vi "Generate Simulated DI Data.vi"(8 "error in":errorcluster, 11 "IONames[]":string[](array[string])) -> (0 "error out":errorcluster, 1 "timestamp":dbl, 2 "data":bool[](array[boolean]))   [LabVIEW 2017, in "DAQ.lvclass"]
doc: "Developed by Kevin Thompson\nkevin@thompsonengineering.net\n\nCopyright 2018-2020\nThompson Engineering, LLC"
uses:
  DAQ.lvclass
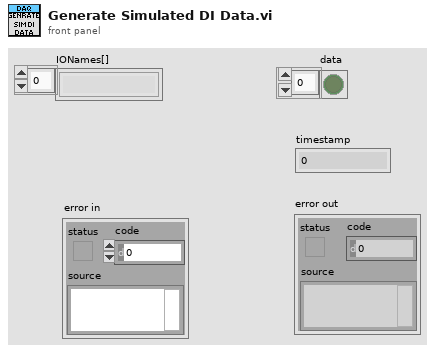
[diagram p1: front panel]
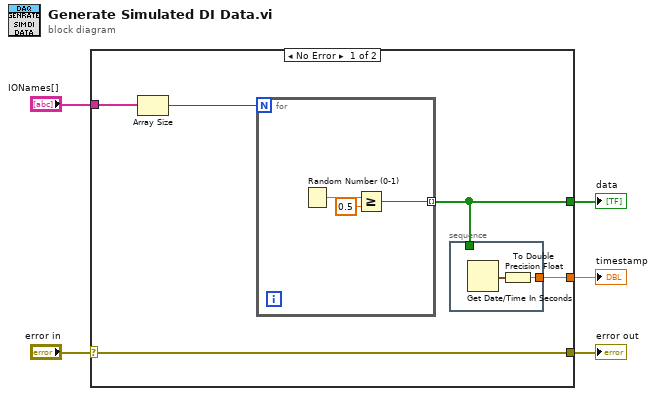
[diagram p0: block diagram]
diagram:
  n1 = case shown="No Error" "error in" {
    selector: "error in" -> [w8 w16]
    tunnel: [w10 _] -> w5
    tunnel: "IONames[]" -> [w9 _]
    tunnel: [w8 w16] -> w2
    tunnel: [w6 _] -> w1
    frame No Error {
      n2 = Array Size(array=w9) -> (size(s)=w7:i32)
      n3 = for {
        N: w7 -> [_]
        tunnel: [w11] -> w6 mode=indexing
        n4 = Random Number (0-1)() -> (number: 0 to 1=w13:dbl)
        n5 = Greater Or Equal?(x=w13, y=0.5) -> (x >= y?=w11:bool)
      }
      n6 = stacked-sequence {
        tunnel: [w14] -> w10
        tunnel: w6 -> [_]
        frame #0 {
          n7 = Get Date/Time In Seconds() -> (seconds since 1Jan1904=w15:timestamp)
          n8 = To Double Precision Float(number=w15) -> (double precision float=w14:dbl)
        }
      }
    }
    frame Error {
    }
  }
  "error out" <- w2
  "data" <- w1
  "timestamp" <- w5
